vi "Check Possible Matches.vi"(7 "Patterns In":bool[][](array[boolean]), 8 "error in (no error)":errorcluster, 10 "ID In":u64, 11 "Tile in":refnum<class "Tile.lvclass">) -> (0 "error out":errorcluster, 3 "Tile out":refnum<class "Tile.lvclass">)   [LabVIEW 2020, in "Tile.lvclass"]
uses:
  Tile.lvclass
  Tile.lvclass/Tile.ctl
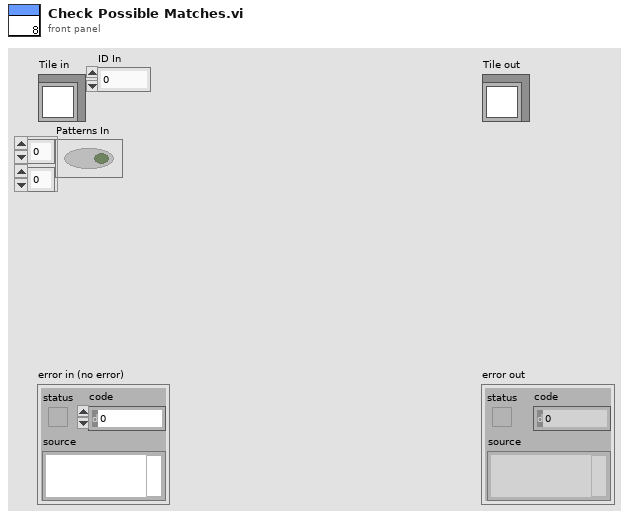
[diagram p1: front panel]
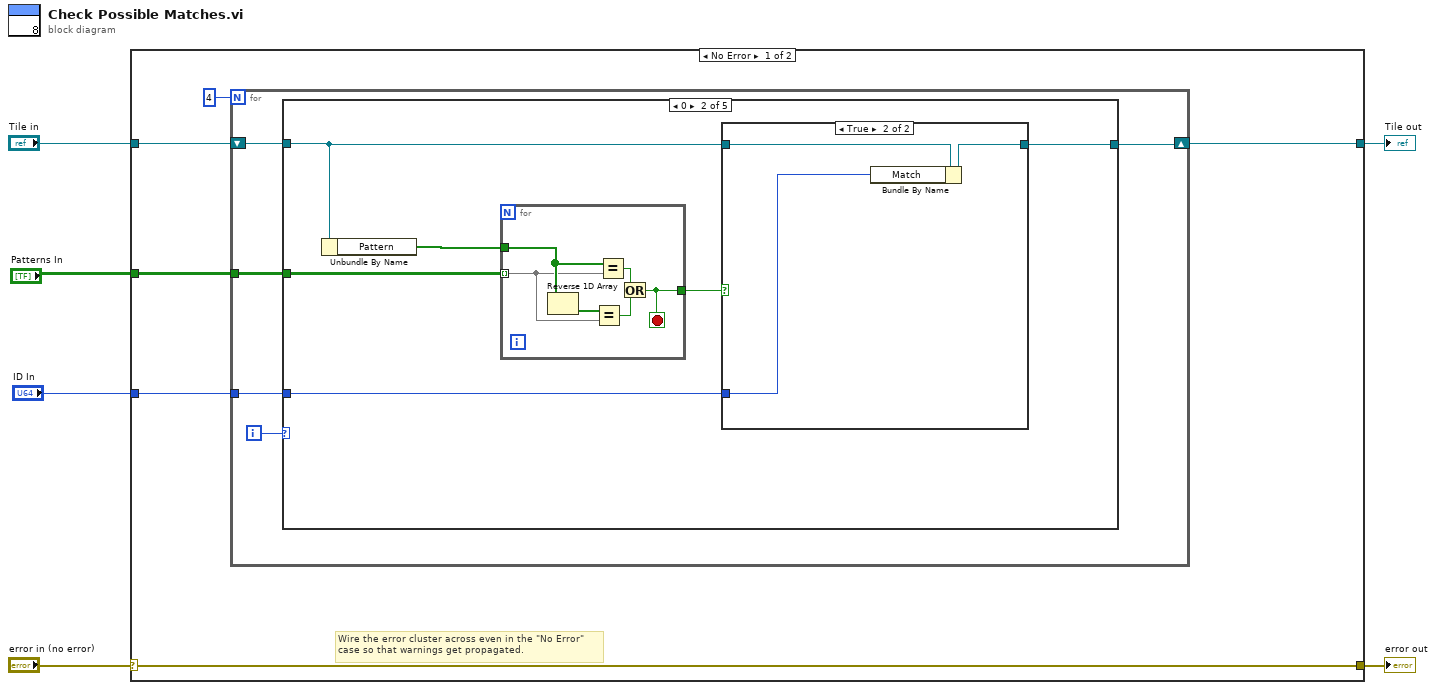
[diagram p0: block diagram]
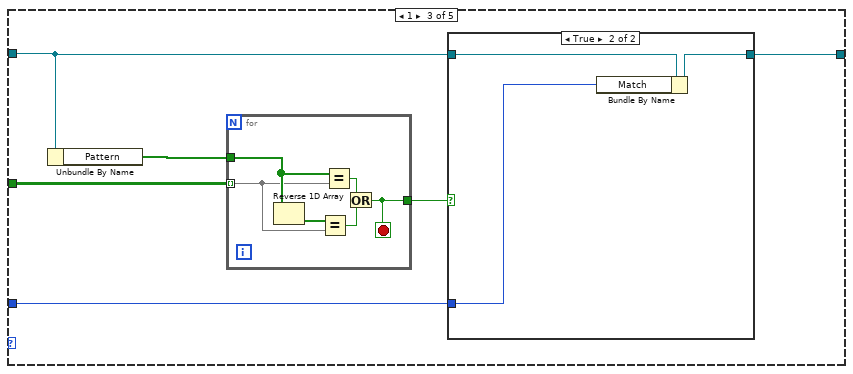
[diagram p4: hidden frame]
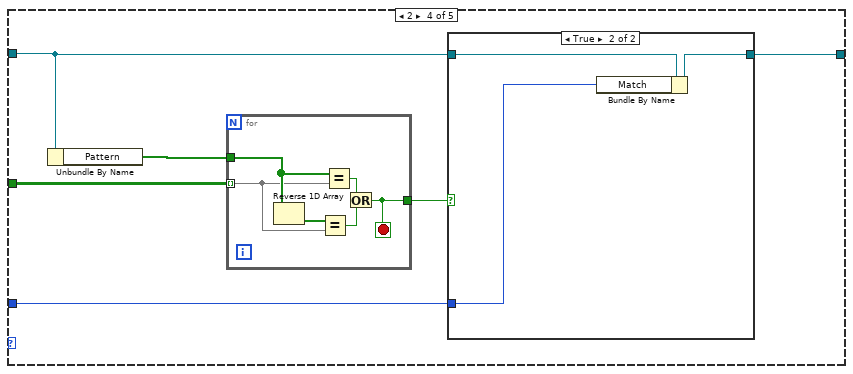
[diagram p6: hidden frame]
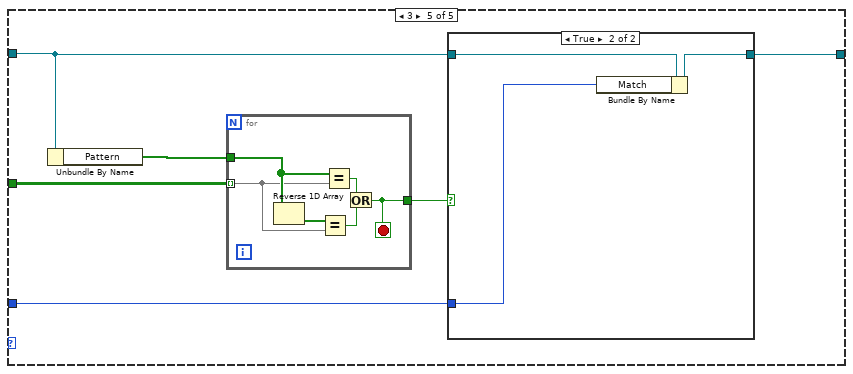
[diagram p8: hidden frame]
diagram:
  n1 = case shown="No Error" "error in (no error)" {
    selector: "error in (no error)" -> [w12 w84]
    tunnel: [w12 w84] -> w5
    tunnel: [w9 w83] -> w3
    tunnel: "Tile in" -> [w8 w83]
    tunnel: "Patterns In" -> [w11 _]
    tunnel: "ID In" -> [w7 _]
    frame No Error {
      # "Wire the error cluster across even in the \"No Error\"\ncase so that warnings get propagated."
      n2 = for {
        N: 4 -> [_]
        tunnel: w11 -> [w17]
        shift-right: [w16] -> w9
        shift-left: w8 -> [w14]
        tunnel: w7 -> [w15]
        i -> [w13]
        n3 = case shown="0" w13 {
          tunnel: w17 -> [_ w24 w40 w56 w72]
          tunnel: [w18 w21 w37 w53 w69] -> w16
          tunnel: w15 -> [_ w20 w36 w52 w68]
          tunnel: w14 -> [w18 w19 w35 w51 w67]
          frame Default {
          }
          frame 0 {
            n4 = Unbundle By Name(w19) -> ("Pattern"=w23:bool[])
            n5 = for {
              tunnel: w24 -> [w29] mode=indexing
              tunnel: w23 -> [w31]
              tunnel: [w30] -> w22
              stop <- w30 stop-if-true
              n6 = Reverse 1D Array(array=w31) -> (reversed array=w32:bool[])
              n7 = Equal?(x=w32, y=w29) -> (x = y?=w33:bool)
              n8 = Equal?(x=w31, y=w29) -> (x = y?=w34:bool)
              n9 = Or(x=w34, y=w33) -> (x .or. y?=w30:bool)
            }
            n10 = case shown="True" w22 {
              tunnel: w19 -> [w25 w28]
              tunnel: [w25 w27] -> w21
              tunnel: w20 -> [_ w26]
              frame False {
              }
              frame True {
                n11 = Bundle By Name(cluster=w28, "Match"=w26) -> (w27:refnum<class "Tile.lvclass">)
              }
            }
          }
          frame 1 {
            n12 = Unbundle By Name(w35) -> ("Pattern"=w39:bool[])
            n13 = for {
              tunnel: w40 -> [w45] mode=indexing
              tunnel: w39 -> [w47]
              tunnel: [w46] -> w38
              stop <- w46 stop-if-true
              n14 = Reverse 1D Array(array=w47) -> (reversed array=w48:bool[])
              n15 = Equal?(x=w48, y=w45) -> (x = y?=w49:bool)
              n16 = Equal?(x=w47, y=w45) -> (x = y?=w50:bool)
              n17 = Or(x=w50, y=w49) -> (x .or. y?=w46:bool)
            }
            n18 = case shown="True" w38 {
              tunnel: w35 -> [w41 w44]
              tunnel: [w41 w43] -> w37
              tunnel: w36 -> [_ w42]
              frame False {
              }
              frame True {
                n19 = Bundle By Name(cluster=w44, "Match"=w42) -> (w43:refnum<class "Tile.lvclass">)
              }
            }
          }
          frame 2 {
            n20 = Unbundle By Name(w51) -> ("Pattern"=w55:bool[])
            n21 = for {
              tunnel: w56 -> [w61] mode=indexing
              tunnel: w55 -> [w63]
              tunnel: [w62] -> w54
              stop <- w62 stop-if-true
              n22 = Reverse 1D Array(array=w63) -> (reversed array=w64:bool[])
              n23 = Equal?(x=w64, y=w61) -> (x = y?=w65:bool)
              n24 = Equal?(x=w63, y=w61) -> (x = y?=w66:bool)
              n25 = Or(x=w66, y=w65) -> (x .or. y?=w62:bool)
            }
            n26 = case shown="True" w54 {
              tunnel: w51 -> [w57 w60]
              tunnel: [w57 w59] -> w53
              tunnel: w52 -> [_ w58]
              frame False {
              }
              frame True {
                n27 = Bundle By Name(cluster=w60, "Match"=w58) -> (w59:refnum<class "Tile.lvclass">)
              }
            }
          }
          frame 3 {
            n28 = Unbundle By Name(w67) -> ("Pattern"=w71:bool[])
            n29 = for {
              tunnel: w72 -> [w77] mode=indexing
              tunnel: w71 -> [w79]
              tunnel: [w78] -> w70
              stop <- w78 stop-if-true
              n30 = Reverse 1D Array(array=w79) -> (reversed array=w80:bool[])
              n31 = Equal?(x=w80, y=w77) -> (x = y?=w81:bool)
              n32 = Equal?(x=w79, y=w77) -> (x = y?=w82:bool)
              n33 = Or(x=w82, y=w81) -> (x .or. y?=w78:bool)
            }
            n34 = case shown="True" w70 {
              tunnel: w67 -> [w73 w76]
              tunnel: [w73 w75] -> w69
              tunnel: w68 -> [_ w74]
              frame False {
              }
              frame True {
                n35 = Bundle By Name(cluster=w76, "Match"=w74) -> (w75:refnum<class "Tile.lvclass">)
              }
            }
          }
        }
      }
    }
    frame Error {
    }
  }
  "error out" <- w5
  "Tile out" <- w3
